vi "Start Async.vi"(8 "error in (no error)":errorcluster, 11 "gRPC Server in":refnum<class "veristand-grpc.lvclass">) -> (0 "error out":errorcluster, 3 "gRPC Server out":refnum<class "veristand-grpc.lvclass">)   [LabVIEW 2021, in "Veristandgrpc_server.lvlib" / "veristand-grpc.lvclass"]
uses:
  veristand-grpc.lvclass
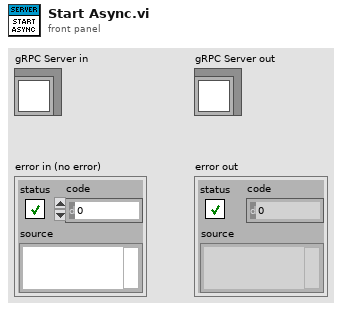
[diagram p1: front panel]
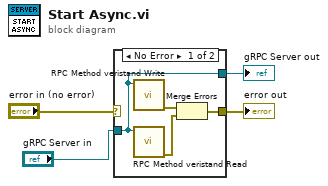
[diagram p0: block diagram]
diagram:
  n1 = case shown="No Error" "error in (no error)" {
    selector: "error in (no error)" -> [_ w10]
    tunnel: [w8 w10] -> w3
    tunnel: [w7 w9] -> w1
    tunnel: "gRPC Server in" -> [w7 w9]
    frame No Error {
      n2 = call "RPC Method veristand Write.vi"("OOP Server in"=w7) -> ("error out"=w6:errorcluster)  [unwired: 9 in, 1 out]
      n3 = call "RPC Method veristand Read.vi"("OOP Server in"=w7) -> ("error out"=w5:errorcluster)  [unwired: 9 in, 1 out]
      n4 = Merge Errors(w6, w5) -> (w8:errorcluster)
    }
    frame Error {
    }
  }
  "error out" <- w3
  "gRPC Server out" <- w1
